vi "Open or Create JSON File.vi"(10 "Application Name":string, 11 "Item Name":string) -> (0 "error out":errorcluster, 3 "JSON File Refnum":refnum<file>)   [LabVIEW 2020, in "JSON File Manipulation.lvlib"]
doc: "Verifica se a pasta, subpastas ou arquivo existem. Se sim, abre arquivo. Se não, cria novo arquivo e popula com a string base."
uses:
  JSON File Manipulation.lvlib
  <vilib>/Utility/sysdir.llb/System Directory Type.ctl
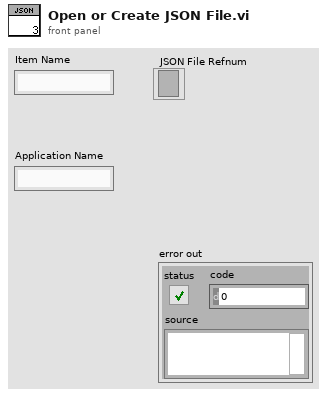
[diagram p1: front panel]
types:
  T1 = typedef "System Directory Type.ctl" = i32
  T2 = enum16{"open", "replace", "create", "open or create", "replace or create", "replace or create with confirmation"}
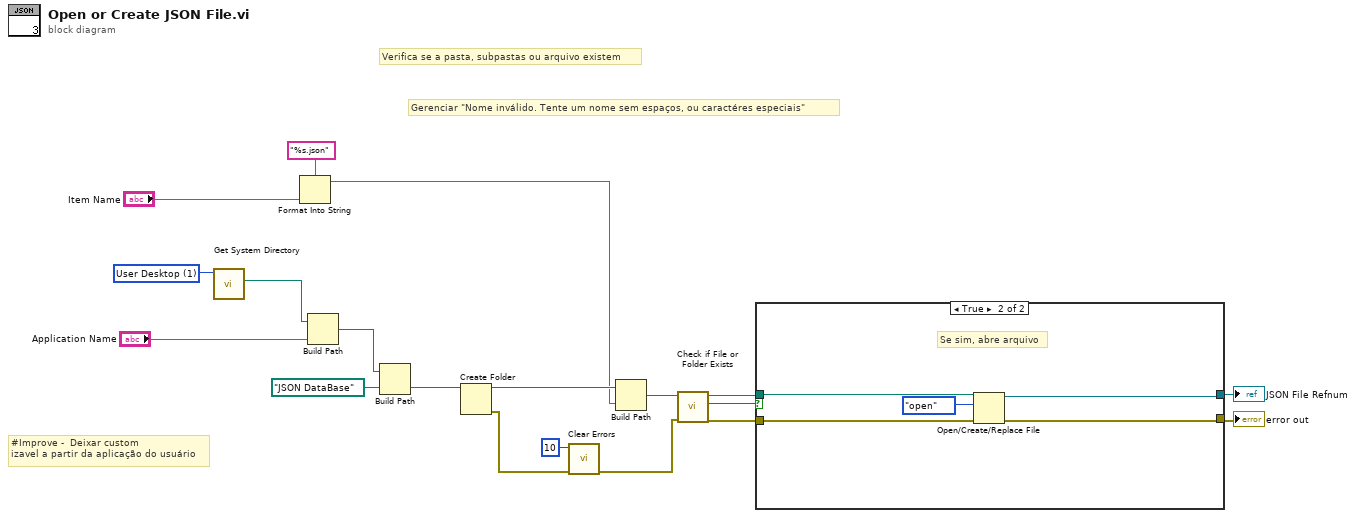
[diagram p0: block diagram]
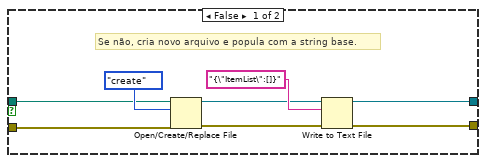
[diagram p2: hidden frame]
diagram:
  w19 = T1 1 items=["User Home"=0, "User Desktop"=1, "User Documents"=2, "User Application Data"=3, "User Preferences"=4, "User Temporary"=5, "Public Documents"=6, "Public Application Data"=7, "Public Preferences"=8, "Public Cache"=13, "System Core Libraries"=9, "System Installed Libraries"=10, "Application Files"=11, "Boot Volume Root"=12] ("system directory type")
  # "Gerenciar \"Nome inválido. Tente um nome sem espaços, ou caractéres especiais\""
  # "#Improve -  Deixar custom\nizavel a partir da aplicação do usuário"
  # "Verifica se a pasta, subpastas ou arquivo existem"
  n1 = call <vilib>:"Get System Directory.vi"("system directory type"=w19) -> ("system directory"=w18:path)  [unwired: 10 in]
  n2 = Format Into String(format string="%s.json", "Item Name") -> (resulting string=w7:string)  [unwired: 2 in, 1 out]
  n3 = Build Path(base path=w18, name or relative path="Application Name") -> (appended path=w3:path)
  n4 = Build Path(base path=w3, name or relative path=path "JSON DataBase") -> (appended path=w4:path)
  n5 = Create Folder(path (use dialog)=w4) -> (created path=w13:path, error out=w12:errorcluster)  [unwired: 2 in, 1 out]
  n6 = call <vilib>:"Clear Errors.vi"("error in (no error)"=w12, "specific error code to clear (0: all)"=10) -> ("error out"=w11:errorcluster)  [unwired: 4 in, 1 out]
  n7 = Build Path(base path=w13, name or relative path=w7) -> (appended path=w17:path)
  n8 = call <vilib>:"Check if File or Folder Exists.vi"("error in (no error)"=w11, "path"=w17) -> ("error out"=w14:errorcluster, "file or folder exists?"=w15:bool, "dup path"=w16:path)  [unwired: 7 in]
  n9 = case shown="True" w15 {
    tunnel: w16 -> [w22 w30]
    tunnel: w14 -> [w26 w32]
    tunnel: [w21 w31] -> w8
    tunnel: [w20 w29] -> w9
    frame False {
      # "Se não, cria novo arquivo e popula com a string base."
      n10 = Open/Create/Replace File(file path (use dialog)=w22, error in=w26, operation (0:open)=T2."create") -> (refnum out=w24:refnum<file>, error out=w23:errorcluster)  [unwired: 3 in, 1 out]
      n11 = Write to Text File(file (use dialog)=w24, text="{\"ItemList\":[]}", error in=w23) -> (refnum out=w20:refnum<file>, error out=w21:errorcluster)  [unwired: 1 in, 1 out]
    }
    frame True {
      # "Se sim, abre arquivo"
      n12 = Open/Create/Replace File(file path (use dialog)=w30, error in=w32, operation (0:open)=T2."open") -> (refnum out=w29:refnum<file>, error out=w31:errorcluster)  [unwired: 3 in, 1 out]
    }
  }
  "JSON File Refnum" <- w9
  "error out" <- w8
